vi "_concat_programmable_mode.vi"(10 "write buffer":string, 11 "Programmable Mode":T1=enum."Basic") -> (2 "write buffer out":string)   [LabVIEW 2023, in "Chemyx_Syringe_Pump_driver.lvlib"]
uses:
  Chemyx_Syringe_Pump_driver.lvlib
  Control/Programmable Mode.ctl
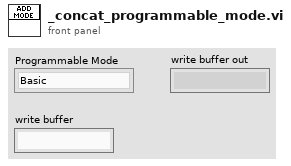
[diagram p1: front panel]
types:
  T1 = typedef "Chemyx_Syringe_Pump_driver.lvlib/Programmable Mode.ctl" = enum16{"Blank", "Basic", "Programmable"}
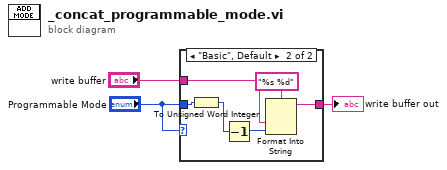
[diagram p0: block diagram]
diagram:
  n1 = case shown="\"Basic\", Default" "Programmable Mode" {
    tunnel: "Programmable Mode" -> [_ w6]
    tunnel: [w4 w10] -> w3
    tunnel: "write buffer" -> [w4 w8]
    frame "Blank" {
    }
    frame "Basic", Default {
      n2 = To Unsigned Word Integer(number=w6) -> (unsigned 16bit integer=w7:u16)
      n3 = Decrement(x=w7) -> (x-1=w5:u16)
      n4 = Format Into String(format string="%s %d", w8, w5) -> (resulting string=w10:string)  [unwired: 2 in, 1 out]
    }
  }
  "write buffer out" <- w3
